vi "Report Duplicate Channels.vi"(7 "Duplicate Channels":string[](array[string]), 8 "error in (no error)":errorcluster) -> (0 "error out":errorcluster)   [LabVIEW 2020, in "Volatus.lvlib" / "VolatusAPI.lvclass"]
uses:
  VolatusAPI.lvclass
  VolatusAPI.lvclass/VolatusAPI.ctl
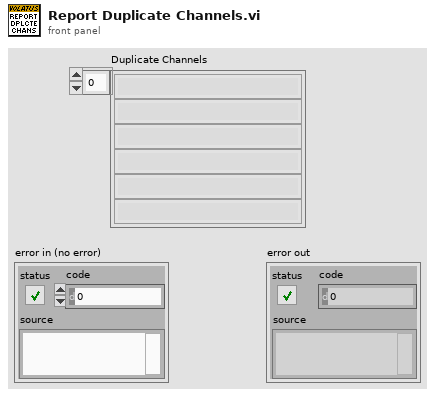
[diagram p1: front panel]
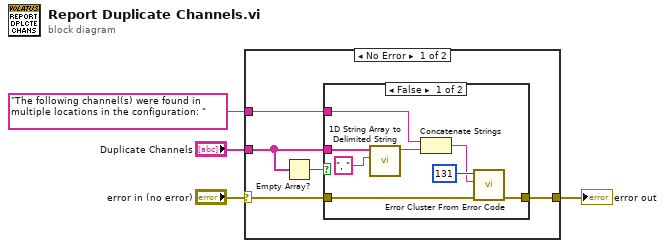
[diagram p0: block diagram]
diagram:
  n1 = case shown="No Error" "error in (no error)" {
    selector: "error in (no error)" -> [w6 w19]
    tunnel: "Duplicate Channels" -> [w8 _]
    tunnel: [w7 w19] -> w2
    tunnel: "The following channel(s) were found in multiple locations in the configuration: " -> [w5 _]
    frame No Error {
      n2 = Empty Array?(array=w8) -> (empty?=w9:bool)
      n3 = case shown="False" w9 {
        tunnel: w8 -> [w14 _]
        tunnel: [w17 w18] -> w7
        tunnel: w6 -> [w16 w18]
        tunnel: w5 -> [w10 _]
        frame False {
          n4 = call <vilib>:"1D String Array to Delimited String.vi"("delimiter"=", ", "string array"=w14) -> ("delimited string"=w12:string)  [unwired: 9 in]
          n5 = Concatenate Strings(w10, w12) -> (w11:string)
          n6 = call <vilib>:"Error Cluster From Error Code.vi"("error in (no error)"=w16, "error message (\"\")"=w11, "error code (0)"=131) -> ("error out"=w17:errorcluster)  [unwired: 6 in]
        }
        frame True {
        }
      }
    }
    frame Error {
    }
  }
  "error out" <- w2
